vi "Target Util.vi"() -> ()   [LabVIEW 2015]
panel:
  out "Center":cluster{"X":dbl, "Y":dbl}
  out "Detected Target":bool
  in  "Points":T1
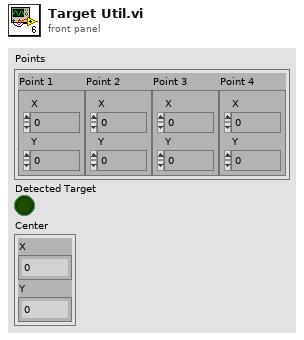
[diagram p1: front panel]
types:
  T1 = cluster{"Point 1":cluster{"X":dbl, "Y":dbl}, "Point 2":cluster{"X":dbl, "Y":dbl}, "Point 3":cluster{"X":dbl, "Y":dbl}, "Point 4":cluster{"X":dbl, "Y":dbl}}
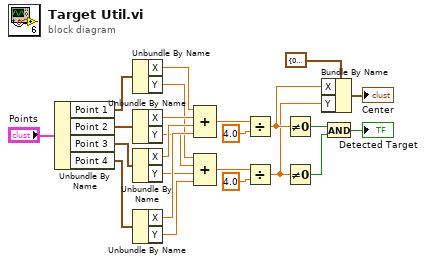
[diagram p0: block diagram]
diagram:
  n1 = Unbundle By Name("Points") -> ("Point 1"=w23:cluster{"X":dbl, "Y":dbl}, "Point 2"=w22:cluster{"X":dbl, "Y":dbl}, "Point 3"=w21:cluster{"X":dbl, "Y":dbl}, "Point 4"=w20:cluster{"X":dbl, "Y":dbl})
  n2 = Unbundle By Name(w23) -> ("X"=w19:dbl, "Y"=w15:dbl)
  n3 = Unbundle By Name(w22) -> ("X"=w18:dbl, "Y"=w14:dbl)
  n4 = Unbundle By Name(w21) -> ("X"=w17:dbl, "Y"=w13:dbl)
  n5 = Unbundle By Name(w20) -> ("X"=w16:dbl, "Y"=w12:dbl)
  n6 = Compound Arithmetic op=ADD(w19, w18, w17, w16) -> (w11:dbl)
  n7 = Compound Arithmetic op=ADD(w15, w14, w13, w12) -> (w8:dbl)
  n8 = Divide(x=w11, y=4.0) -> (x/y=w6:dbl)
  n9 = Divide(x=w8, y=4.0) -> (x/y=w5:dbl)
  n10 = Not Equal To 0?(x=w6) -> (x != 0?=w3:bool)
  n11 = Not Equal To 0?(x=w5) -> (x != 0?=w4:bool)
  n12 = Bundle By Name(cluster=cluster{"X":dbl, "Y":dbl} {"X"=0.0, "Y"=0.0} ("Point 1"), "X"=w6, "Y"=w5) -> (→"Center":cluster{"X":dbl, "Y":dbl})
  n13 = And(x=w3, y=w4) -> (x .and. y?=→"Detected Target":bool)
